vi "Write Handle.vi"(8 "error in (no error)":errorcluster, 10 "Handle":i16, 11 "PicoScope 3000a in":refnum<class "PicoScope 3000a.lvclass">) -> (0 "error out":errorcluster, 3 "PicoScope 3000a out":refnum<class "PicoScope 3000a.lvclass">)   [LabVIEW 2018, in "PicoScope 3000a.lvlib" / "PicoScope 3000a.lvclass"]
uses:
  PicoScope 3000a.lvclass
  PicoScope 3000a.lvclass/PicoScope 3000a.ctl
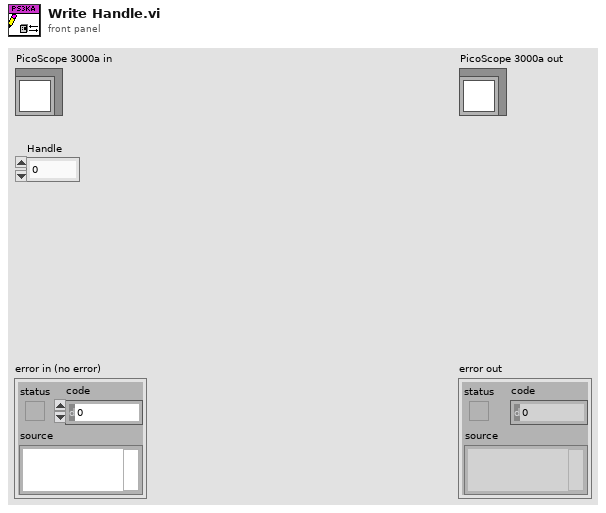
[diagram p1: front panel]
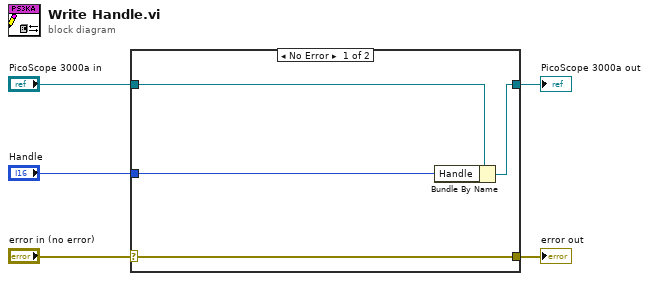
[diagram p0: block diagram]
diagram:
  n1 = case shown="No Error" "error in (no error)" {
    selector: "error in (no error)" -> [w9 w10]
    tunnel: [w9 w10] -> w4
    tunnel: [w7 w11] -> w2
    tunnel: "PicoScope 3000a in" -> [w8 w11]
    tunnel: "Handle" -> [w6 _]
    frame No Error {
      n2 = Bundle By Name(cluster=w8, "Handle"=w6) -> (w7:refnum<class "PicoScope 3000a.lvclass">)
    }
    frame Error {
    }
  }
  "error out" <- w4
  "PicoScope 3000a out" <- w2
